vi "Globals.vi"() -> ()   [LabVIEW 2017, in "nifxpmath_Exp.xnode"]
uses:
  <vilib>/rvi/FXPMathLib/FxpExp/XNode/nifxpmath_Exp.xnode
panel:
  out "SMALLICON w/ 4WIRE":picture
  in  "Term E Name":string="exp(x)"
  in  "Term Z Name":string="x"
  out "SMALLICON":picture
  out "NORMALBANNER":picture
  in  "Term E ID":string="TERM_E"
  in  "Term Z ID":string="TERM_Z"
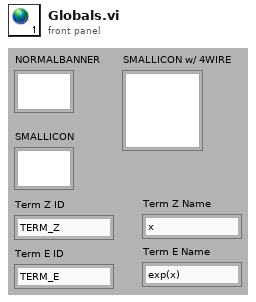
[diagram p1: front panel]
diagram:
